vi "Engine-RPC-IMVCtrl.vi"(0 "Control Enable":bool, 1 "Fault Input":bool, 2 "Rail Press Setpoint":sgl format="%.2f", 3 "Rail Pressure":sgl format="%.2f", 5 "PID Enable":bool, 9 "PID Settings":T5={"PID_Kp"=0.0, "PID_Ti"=0.01, "PID_Td"=0.0, "PID_FF"=0.0, "Non-PID_FF"=0.0, "PID_Min"=-100.0, "PID_Max"=100.0} {"PID_Max" format="%.2f"; "PID_Min" format="%.2f"; "PID_Td" format="%.3f"; "PID_Ti" format="%.3f"}, 11 "Output Management Controls":T4, 12 "dt (s)":sgl=-1.0 format="%.3f", 13 "Battery [V]":sgl) -> (4 "Output":T1={"Current_Calc"=0.0, "DutyCyc_PIDOut"=0.7671859, "DutyCyc_MaxCalc"=0.0, "DutyCyc_Des"=0.7671859}, 14 "PID_Action_Output":T3, 15 "LS Output":T2)   [LabVIEW 2016, in "DSI-RT.lvlib"]
uses:
  DSI-RT.lvlib
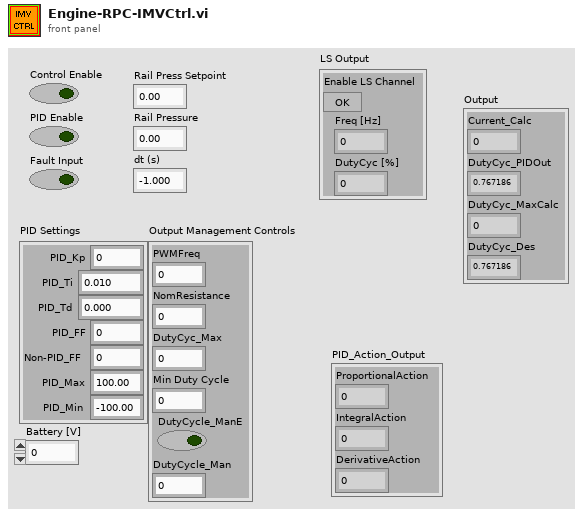
[diagram p1: front panel]
types:
  T1 = cluster{"Current_Calc":sgl, "DutyCyc_PIDOut":sgl, "DutyCyc_MaxCalc":sgl, "DutyCyc_Des":sgl}
  T2 = cluster{"Enable LS Channel":bool, "Freq [Hz]":sgl, "DutyCyc [%]":sgl}
  T3 = cluster{"ProportionalAction":sgl, "IntegralAction":sgl, "DerivativeAction":sgl}
  T4 = cluster{"PWMFreq":sgl, "NomResistance":sgl, "DutyCyc_Max":sgl, "Min Duty Cycle":sgl, "DutyCycle_ManE":bool, "DutyCycle_Man":sgl}
  T5 = cluster{"PID_Kp":sgl, "PID_Ti":sgl, "PID_Td":sgl, "PID_FF":sgl, "Non-PID_FF":sgl, "PID_Min":sgl, "PID_Max":sgl}
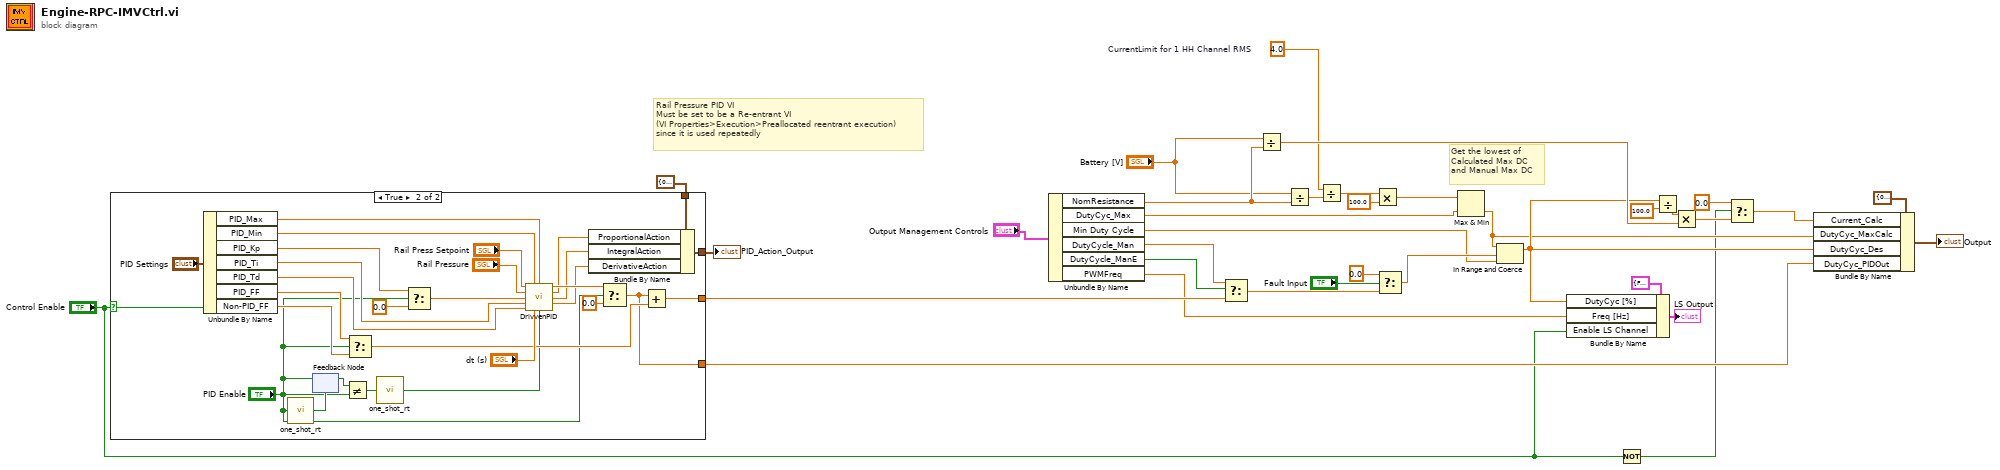
[diagram p0: block diagram]
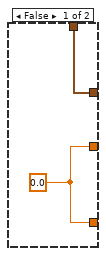
[diagram p2: hidden frame]
diagram:
  w7 = sgl 4.0  # CurrentLimit for 1 HH Channel RMS
  # "Rail Pressure PID VI\nMust be set to be a Re-entrant VI \n(VI Properties>Execution>Preallocated reentrant execution)\nsince it is used repeatedly"
  # "Get the lowest of \nCalculated Max DC\nand Manual Max DC"
  n1 = case shown="True" "Control Enable" {
    tunnel: [w37 w57] -> w21
    tunnel: [w37 w54] -> w23
    tunnel: T3 {"ProportionalAction"=0.0, "IntegralAction"=0.0, "DerivativeAction"=0.0} -> [w36 w43]
    tunnel: [w36 w42] -> w13
    frame False {
      w37 = sgl 0.0 ("f")
    }
    frame True {
      n2 = Unbundle By Name("PID Settings") -> ("PID_Max"=w50:sgl, "PID_Min"=w49:sgl, "PID_Kp"=w51:sgl, "PID_Ti"=w48:sgl, "PID_Td"=w47:sgl, "PID_FF"=w46:sgl, "Non-PID_FF"=w45:sgl)
      n3 = call <vilib>:"one_shot_rt.vi"("I"="PID Enable") -> ("O"=w39:bool)
      n4 = feedback #1(w39) -> (w56:bool)
      n5 = feedback-in #1("PID Enable") -> ()
      n6 = Not Equal?(x=w56, y="PID Enable") -> (x != y?=w55:bool)
      n7 = Select(t=w46, s="PID Enable", f=w45) -> (s? t:f=w60:sgl)
      n8 = call <vilib>:"one_shot_rt.vi"("I"=w55) -> ("O"=w53:bool)
      n9 = Select(t=w51, s="PID Enable", f=sgl 0.0 ("t")) -> (s? t:f=w64:sgl)
      n10 = call <vilib>:"DrivvenPID.vi"("Setpoint"="Rail Press Setpoint", "OutputLow"=w49, "OutputHigh"=w50, "ProcessVariable"="Rail Pressure", "ProportionalGain (Kc)"=w64, "IntegralTime (Ti, min)"=w48, "DerivativeTime (Td, min)"=w47, "dt (s)"="dt (s)", "Reinitialize? (F)"=w53) -> ("Output"=w59:sgl, "ProportionalAction"=w44:sgl, "IntegralAction"=w41:sgl, "DerivativeAction"=w40:sgl)  [unwired: 1 in, 2 out]
      n11 = Bundle By Name(cluster=w43, "ProportionalAction"=w44, "IntegralAction"=w41, "DerivativeAction"=w40) -> (w42:T3)
      n12 = Select(t=w59, s="PID Enable", f=sgl 0.0) -> (s? t:f=w57:sgl)
      n13 = Add(x=w57, y=w60) -> (x+y=w54:sgl)
    }
  }
  "PID_Action_Output" <- w13
  n14 = Unbundle By Name("Output Management Controls") -> ("NomResistance"=w11:sgl, "DutyCyc_Max"=w9:sgl, "Min Duty Cycle"=w19:sgl, "DutyCycle_Man"=w18:sgl, "DutyCycle_ManE"=w17:bool, "PWMFreq"=w15:sgl)
  n15 = Select(t=w18, s=w17, f=w23) -> (s? t:f=w25:sgl)
  n16 = Divide(x="Battery [V]", y=w11) -> (x/y=w32:sgl)
  n17 = Divide(x="Battery [V]", y=w11) -> (x/y=w31:sgl)
  n18 = Divide(x=w7, y=w31) -> (x/y=w30:sgl)
  n19 = Multiply(x=w30, y=sgl 100.0) -> (x*y=w10:sgl)
  n20 = Select(t=sgl 0.0, s="Fault Input", f=w25) -> (s? t:f=w24:sgl)
  n21 = Max & Min(x=w10, y=w9) -> (min(x,y)=w8:sgl)  [unwired: 1 out]
  n22 = In Range and Coerce(upper limit=w8, x=w24, lower limit=w19) -> (coerced(x)=w16:sgl)  [unwired: 1 out]
  n23 = Bundle By Name(cluster=T2 {"Enable LS Channel"=FALSE, "Freq [Hz]"=0.0, "DutyCyc [%]"=0.0} ("LS Output"), "DutyCyc [%]"=w16, "Freq [Hz]"=w15, "Enable LS Channel"="Control Enable") -> (→"LS Output":T2)
  n24 = Not(x="Control Enable") -> (.not. x?=w4:bool)
  n25 = Divide(x=w16, y=sgl 100.0) -> (x/y=w33:sgl)
  n26 = Multiply(x=w33, y=w32) -> (x*y=w35:sgl)
  n27 = Select(t=sgl 0.0, s=w4, f=w35) -> (s? t:f=w22:sgl)
  n28 = Bundle By Name(cluster=T1 {"Current_Calc"=0.0, "DutyCyc_PIDOut"=0.7671859, "DutyCyc_MaxCalc"=0.0, "DutyCyc_Des"=0.7671859} ("IMV 2"), "Current_Calc"=w22, "DutyCyc_MaxCalc"=w8, "DutyCyc_Des"=w16, "DutyCyc_PIDOut"=w21) -> (→"Output":T1)
